vi "Read Sub panel coin.vi"(8 "error in (no error)":errorcluster, 11 "USD ACTOR in":refnum<class "USD ACTOR.lvclass">) -> (0 "error out":errorcluster, 2 "Sub panel coin":refnum<vi>, 3 "USD ACTOR out":refnum<class "USD ACTOR.lvclass">)   [LabVIEW 2019, in "USD ACTOR.lvlib" / "USD ACTOR.lvclass"]
uses:
  USD ACTOR.lvclass
  USD ACTOR.lvclass/USD ACTOR.ctl
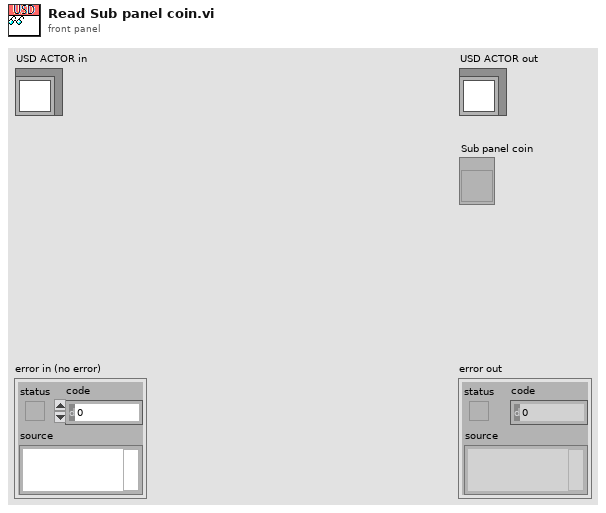
[diagram p1: front panel]
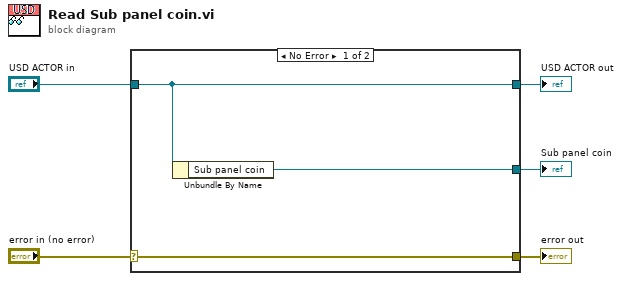
[diagram p0: block diagram]
diagram:
  n1 = case shown="No Error" "error in (no error)" {
    selector: "error in (no error)" -> [w8 w9]
    tunnel: [w8 w9] -> w4
    tunnel: [w7 w10] -> w2
    tunnel: "USD ACTOR in" -> [w7 w10]
    tunnel: [w6 _] -> w1
    frame No Error {
      n2 = Unbundle By Name(w7) -> ("Sub panel coin"=w6:refnum<vi>)
    }
    frame Error {
    }
  }
  "error out" <- w4
  "USD ACTOR out" <- w2
  "Sub panel coin" <- w1
